vi "Get Options.vi"(8 "error in (no error)":errorcluster, 11 "Shared Options in":refnum<class "Shared Options.lvclass">) -> (0 "error out":errorcluster, 2 "Options":string[](array[string]), 3 "Shared Options out":refnum<class "Shared Options.lvclass">)   [LabVIEW 2020, in "AutoComplete.lvlib" / "Shared Options.lvclass"]
uses:
  Shared Options.lvclass
  Shared Options.lvclass/Shared Options.ctl
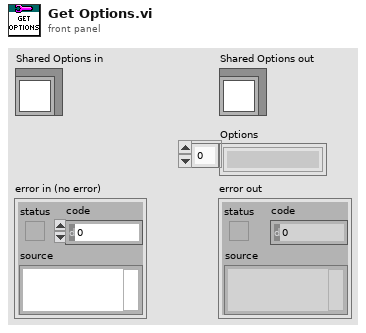
[diagram p1: front panel]
types:
  T1 = typedef "AutoComplete.lvlib/Options.ctl" = cluster{"Options":string[], "Allow Undefined Values":bool}
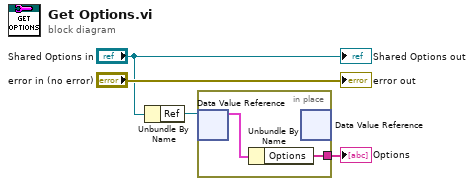
[diagram p0: block diagram]
diagram:
  n1 = Unbundle By Name("Shared Options in") -> ("Ref"=w2:refnum<data-value>)
  n2 = in-place {
    in-place-border: [w5] -> w1
    n3 = in-place-dvr #1(w2) -> (w6:T1)  [unwired: 1 out]
    n4 = Unbundle By Name(w6) -> ("Options"=w5:string[])
    n5 = in-place-dvr #1() -> ()  [unwired: 1 in, 2 out]
  }
  "Options" <- w1
  "error out" <- "error in (no error)"
  "Shared Options out" <- "Shared Options in"
